vi "db_connect.vi"() -> ()   [LabVIEW 2016]
uses:
  <vilib>/addons/database/Connection.llb/DB Tools Open Connec (Path).vi
  <vilib>/addons/database/_DB Variant To Data/Database Variant To Data.xnode
  <vilib>/addons/database/NI_Database_API.lvlib
panel:
  in  "Data":T1
  in  "Novo":bool
  in  "input 1":dbl=9.0
  out "data 2":string[][](array[string])
  out "subarray":string[](array[string])
  in  "stop":bool
  out "data":string[][](array[string])=[["1", "Bateria Unipower 1", "12", "7"], ["2", "Bateria Unipower 2", "12", "7"], ["3", "Bateria Unipower 3", "12", "7"], ["4", "Bateria Unipower 4", "12", "7"], ["5", "Bateria Unipower 5", "12", "7"], ["6", "Bateria Unipower 6", "12", "7"], ["7", "Bateria Unipower 7", "12", "7"], ["8", "Bateria Unipower 8", "12", "7"]]
  in  "connection information":path=path "D:/UFSM/Engenharia de Controle e Automação/8 Semestre/Projeto Integrador - DPEE 1064/LabVIEW/database.udl"
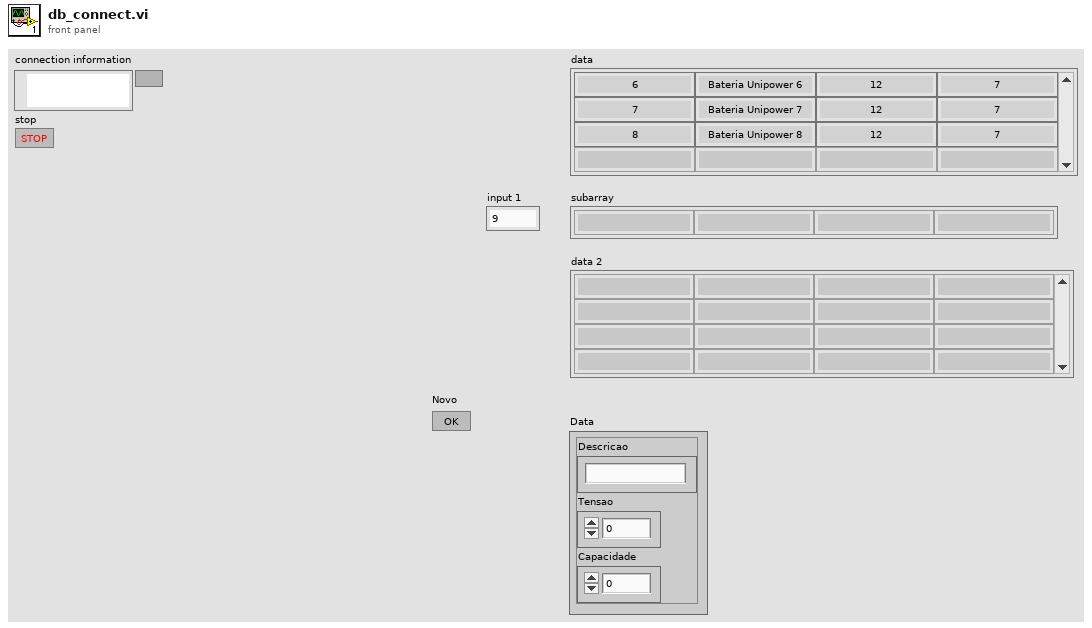
[diagram p1: front panel]
types:
  T1 = cluster{"Descricao":string, "Tensao":i32, "Capacidade":i32}
  T2 = typedef "NI_Database_API.lvlib/Conn ObjectReference.ctl" = refnum<k1>
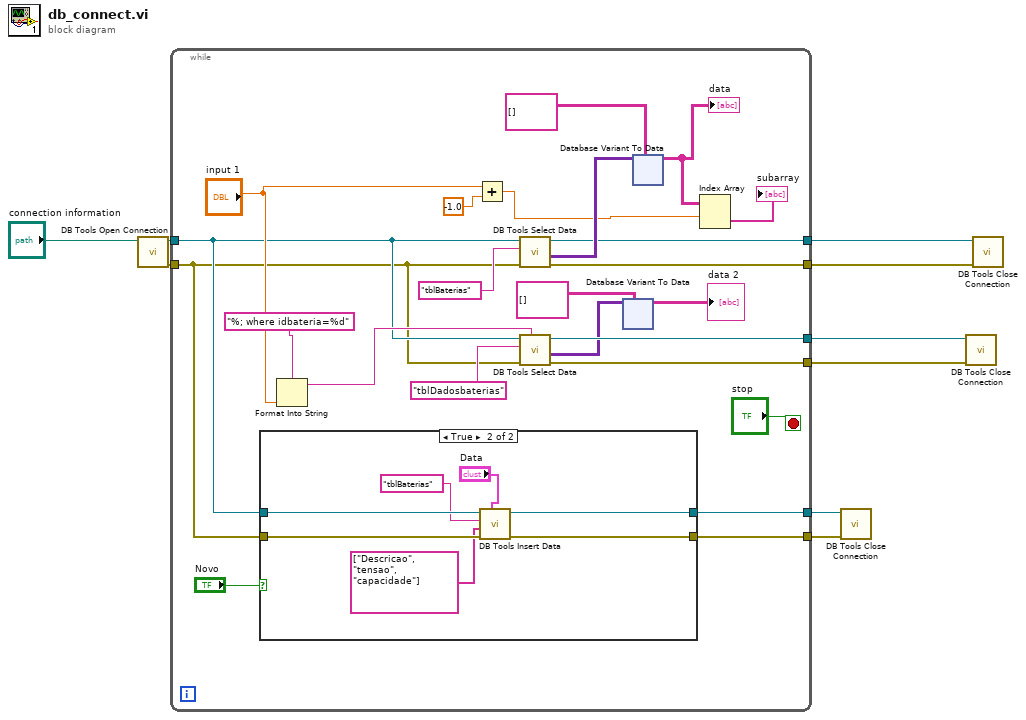
[diagram p0: block diagram]
diagram:
  n1 = call-poly <vilib>:"DB Tools Open Connection.vi"("connection information"="connection information") -> ("error out"=w8:errorcluster, "connection reference"=w5:T2)  [unwired: 7 in]
  n2 = while {
    tunnel: w8 -> [w13]
    tunnel: [w27] -> w7
    tunnel: [w26] -> w6
    tunnel: w5 -> [w16]
    tunnel: [w15] -> w4
    tunnel: [w14] -> w3
    tunnel: [w12] -> w2
    tunnel: [w11] -> w1
    stop <- "stop" stop-if-true
    n3 = case shown="True" "Novo" {
      tunnel: w16 -> [w35 w42]
      tunnel: w13 -> [w34 w41]
      tunnel: [w35 w40] -> w12
      tunnel: [w34 w39] -> w11
      frame False {
      }
      frame True {
        n4 = call <vilib>:"DB Tools Insert Data.vi"("data"="Data", "error in (no error)"=w41, "columns"=string[] ["Descricao", "tensao", "capacidade"], "table"="tblBaterias", "connection reference"=w42) -> ("error out"=w39:errorcluster, "connection reference out"=w40:T2)  [unwired: 5 in]
      }
    }
    n5 = Format Into String(format string="%; where idbateria=%d" ("condition"), "input 1") -> (resulting string=w17:string)  [unwired: 2 in, 1 out]
    n6 = Add(x="input 1", y=-1.0) -> (x+y=w19:dbl)
    n7 = call <vilib>:"DB Tools Select Data.vi"("error in (no error)"=w13, "table"="tblBaterias", "connection reference"=w16) -> ("error out"=w14:errorcluster, "data"=w32:variant[][], "connection reference out"=w15:T2)  [unwired: 3 in]
    n8 = call <vilib>:"DB Tools Select Data.vi"("condition"=w17, "error in (no error)"=w13, "table"="tblDadosbaterias", "connection reference"=w16) -> ("error out"=w26:errorcluster, "data"=w25:variant[][], "connection reference out"=w27:T2)  [unwired: 2 in]
    n9 = xnode "Database Variant To Data"("database variant"=w25, "type"=string[][] []) -> ("data"=→"data 2":string[][])  [unwired: 1 in, 1 out]
    n10 = xnode "Database Variant To Data"("database variant"=w32, "type"=string[][] []) -> ("data"=w29:string[][])  [unwired: 1 in, 1 out]
    "data" <- w29
    n11 = Index Array(array=w29, index (row)=w19) -> (element=→"subarray":string[])  [unwired: 1 in]
  }
  n12 = call <vilib>:"DB Tools Close Connection.vi"("error in (no error)"=w1, "connection reference"=w2) -> ()  [unwired: 5 in, 1 out]
  n13 = call <vilib>:"DB Tools Close Connection.vi"("error in (no error)"=w6, "connection reference"=w7) -> ()  [unwired: 5 in, 1 out]
  n14 = call <vilib>:"DB Tools Close Connection.vi"("error in (no error)"=w3, "connection reference"=w4) -> ()  [unwired: 5 in, 1 out]
